vi "EXA1.vi"(11 "Variables and Memory in":T1 {"GFX" format="%02x"}) -> (3 "Variables and Memory out":T1 {"GFX" format="%02x"})   [LabVIEW 2021]
uses:
  Controls/ClusterF.ctl
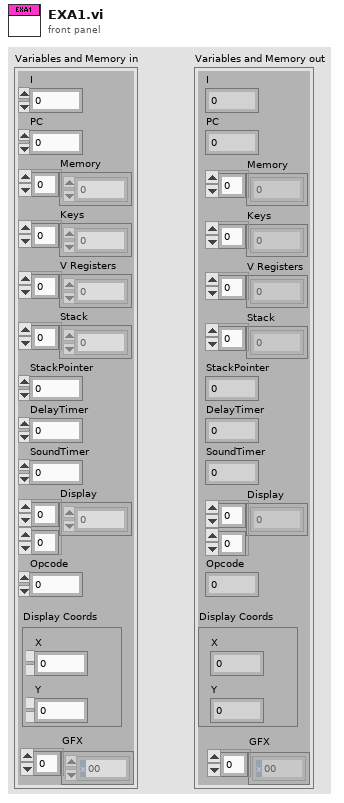
[diagram p1: front panel]
types:
  T1 = typedef "ClusterF.ctl" = cluster{"I":u16, "PC":u16, "Memory":u8[], "Keys":u8[], "V Registers":u8[], "Stack":u16[], "StackPointer":u16, "DelayTimer":u8, "SoundTimer":u8, "Display":u8[][], "Opcode":u16, "Display Coords":cluster{"X":u8, "Y":u8}, "GFX":u8[]}
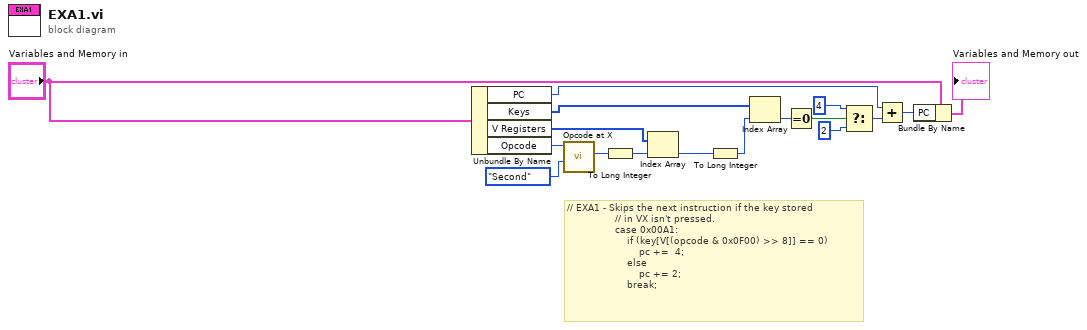
[diagram p0: block diagram]
diagram:
  # "// EXA1 - Skips the next instruction if the key stored\n                // in VX isn't pressed.\n                case 0x00A1:\n                    if (key[V[(opcode & 0x0F00) >> 8]] == 0)\n                        pc +=  4;\n                    else\n                        pc += 2;\n                    break;"
  n1 = Unbundle By Name("Variables and Memory in") -> ("PC"=w2:u16, "Keys"=w7:u8[], "V Registers"=w6:u8[], "Opcode"=w17:u16)
  n2 = call "Opcode at X.vi"("X Position"=enum16{"First", "Second", "Third", "Fourth"}."Second", "Opcode"=w17) -> ("Opcode at X Position (U8)"=w12:u8)  [unwired: 9 in]
  n3 = To Long Integer(number=w12) -> (32bit integer=w11:i32)
  n4 = Index Array(array=w6, index=w11) -> (element=w9:u8)
  n5 = To Long Integer(number=w9) -> (32bit integer=w10:i32)
  n6 = Index Array(array=w7, index=w10) -> (element=w8:u8)
  n7 = Equal To 0?(x=w8) -> (x = 0?=w15:bool)
  n8 = Select(t=u16 4 ("y"), s=w15, f=u16 2 ("y")) -> (s? t:f=w16:u16)
  n9 = Add(x=w2, y=w16) -> (x+y=w5:u16)
  n10 = Bundle By Name(cluster="Variables and Memory in", "PC"=w5) -> (→"Variables and Memory out":T1)
